vi "Call Msg Send.vi"(7 "LVCAM":refnum<class "LVCAM.lvclass">, 9 "Priority?":bool, 10 "Msg":refnum<class "Msg.lvclass">) -> (0 "error out":errorcluster)   [LabVIEW 2021, in "LVCAM.lvlib" / "Self Actor.lvclass"]
uses:
  Self Actor.lvclass
  Msg/Msg.lvclass
  LVCAM/LVCAM.lvclass
  Self Actor.lvclass/Self Actor.ctl
  Msg Q/Msg Q.lvclass
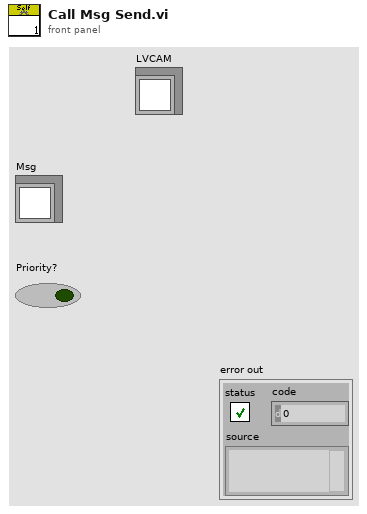
[diagram p1: front panel]
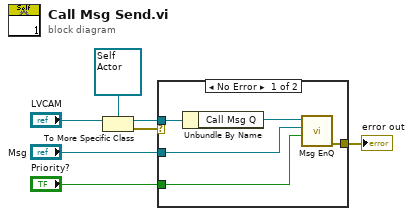
[diagram p0: block diagram]
diagram:
  n1 = To More Specific Class(target class=refnum<class "Self Actor.lvclass"> refnum ("LVCAM.lvlib:Self Actor.lvclass"), reference="LVCAM") -> (specific class reference=w3:refnum<class "Self Actor.lvclass">, error out=w1:errorcluster)  [unwired: 1 in]
  n2 = case shown="No Error" w1 {
    selector: w1 -> [_ w13]
    tunnel: "Msg" -> [w11 _]
    tunnel: [w10 w13] -> w6
    tunnel: "Priority?" -> [w9 _]
    tunnel: w3 -> [w8 _]
    frame No Error {
      n3 = Unbundle By Name(w8) -> ("Call Msg Q"=w12:refnum<class "Msg Q.lvclass">)
      n4 = call "Msg EnQ.vi"("Priority?"=w9, "Msg"=w11, "Msg Q in"=w12) -> ("error out"=w10:errorcluster)  [unwired: 8 in]
    }
    frame Error {
    }
  }
  "error out" <- w6
